vi "Define Name.vi"(8 "error in":errorcluster, 11 "NI 9474 in":refnum<class "NI 9474.lvclass">) -> (0 "error out":errorcluster, 3 "NI 9474 out":refnum<class "NI 9474.lvclass">)   [LabVIEW 2017, in "Scan Engine Scripting.lvlib" / "NI 9474.lvclass"]
uses:
  NI 9474.lvclass
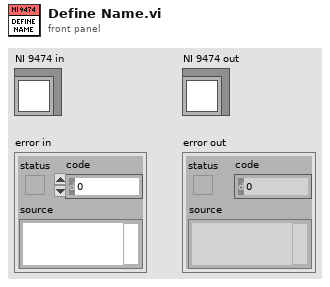
[diagram p1: front panel]
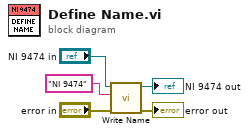
[diagram p0: block diagram]
diagram:
  n1 = call-dynamic "Write Name.vi"("error in"="error in", "name"="NI 9474", "module in"="NI 9474 in") -> ("error out"=→"error out":errorcluster, "module out"=→"NI 9474 out":refnum<class "NI 9474.lvclass">)  [unwired: 7 in]
